vi "changeSessionLabbookHelpervi.vi"(8 "strControlText":string, 10 "error in (no error)":errorcluster) -> (2 "error out":errorcluster)   [LabVIEW 2014]
panel:
  in  "AutoItX3Lib.IAutoItX3":refnum<k7>
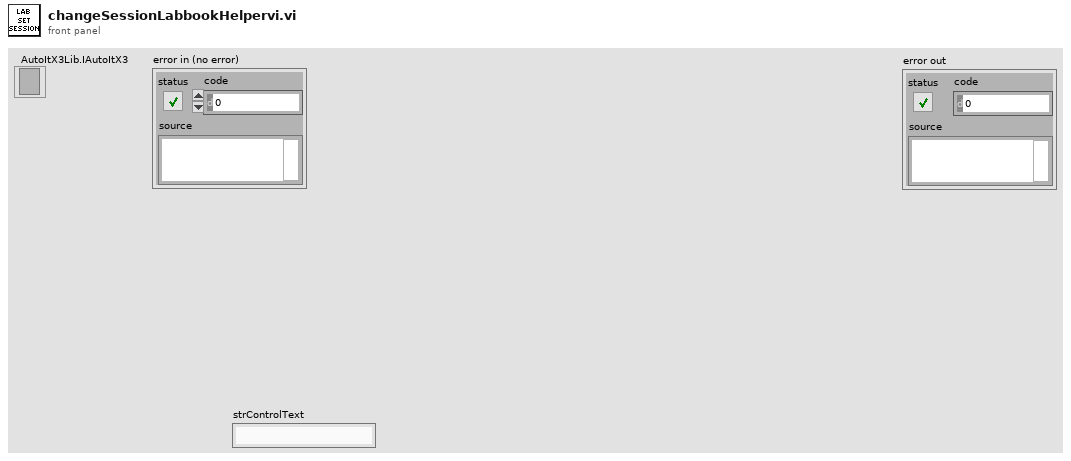
[diagram p1: front panel]
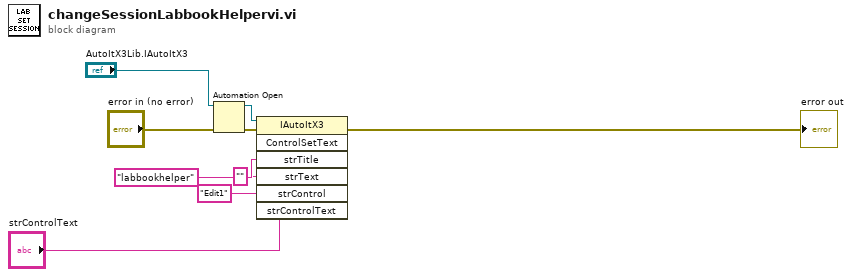
[diagram p0: block diagram]
diagram:
  n1 = Automation Open(error in (no error)="error in (no error)", Automation Refnum="AutoItX3Lib.IAutoItX3") -> (Automation Refnum=w7:refnum<k7>, error out=w8:errorcluster)  [unwired: 2 in]
  n2 = invoke class="IAutoItX3" method="ControlSetText"(reference=w7, error in=w8, "strTitle"="labbookhelper", "strText"="", "strControl"="Edit1", "strControlText"="strControlText") -> (error out=→"error out":errorcluster)  [unwired: 1 in, 6 out]
